vi "MenuActive(Data).vi"(8 "error in (no error)":errorcluster caption="错误输入（无错误）", 10 "菜单引用":refnum<k9>, 11 "PanelDataNode 输入":refnum<class "PanelDataNode.lvclass"> caption="DNL_LabVIEW Object in") -> (0 "error out":errorcluster caption="错误输出", 2 "menu reference out":refnum<k9>, 3 "PanelDataNode 输出":refnum<class "PanelDataNode.lvclass"> caption="DNL_LabVIEW Object out")   [LabVIEW 2013, in "PanelDataNode.lvclass"]
uses:
  PanelDataNode.lvclass
  PanelDataNode.lvclass/PanelDataNode.ctl
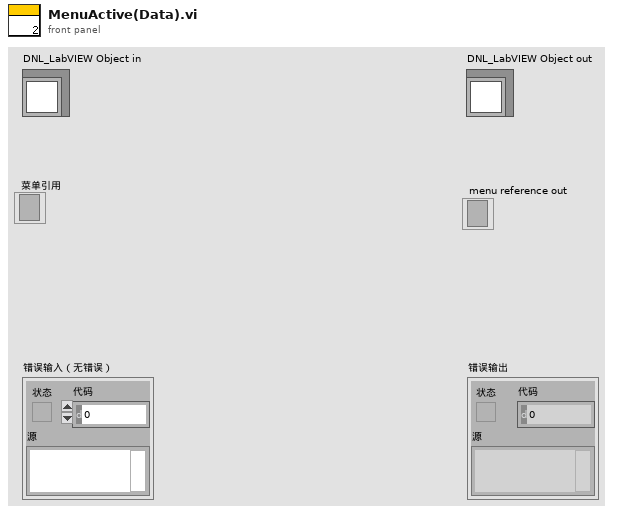
[diagram p1: front panel]
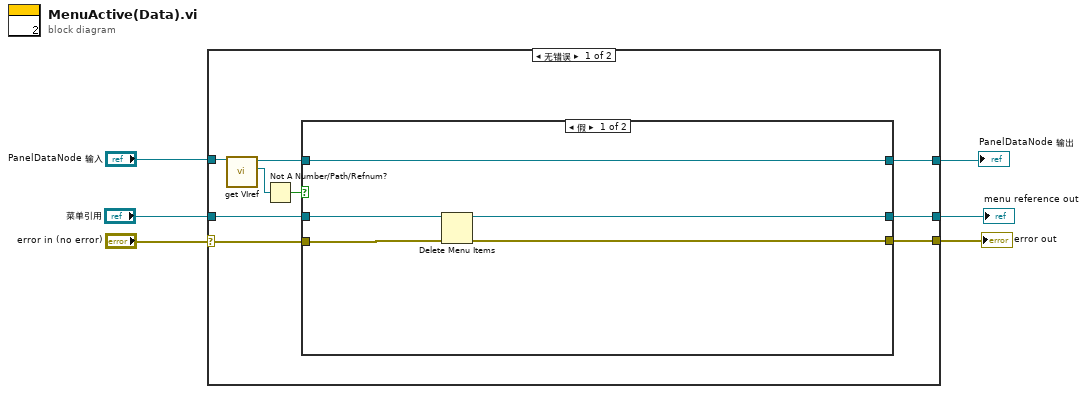
[diagram p0: block diagram]
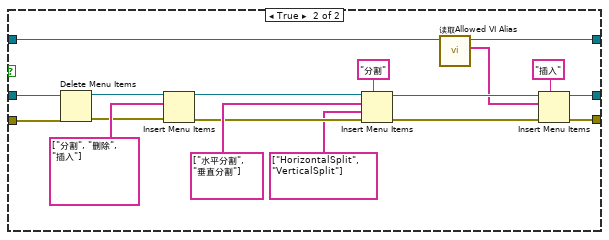
[diagram p2: hidden frame]
diagram:
  n1 = case shown="无错误" "error in (no error)" {
    selector: "error in (no error)" -> [w13 w41]
    tunnel: [w14 w40] -> w5
    tunnel: [w15 w41] -> w4
    tunnel: "PanelDataNode 输入" -> [w10 w40]
    tunnel: "菜单引用" -> [w9 w39]
    tunnel: [w8 w39] -> w1
    frame No Error {
      n2 = call "get VIref.vi"("PanelDataNode输入"=w10) -> ("VI*"=w7:refnum<vi>, "PanelDataNode输出"=w12:refnum<class "PanelDataNode.lvclass">)  [unwired: 8 in, 1 out]
      n3 = Not A Number/Path/Refnum?(number/path/refnum=w7) -> (NaN/Path/Refnum?=w11:bool)
      n4 = case shown="假" w11 {
        tunnel: [w17 w29] -> w15
        tunnel: w12 -> [w20 w27]
        tunnel: [w20 w25] -> w14
        tunnel: w13 -> [w18 w23]
        tunnel: w9 -> [w19 w22]
        tunnel: [w16 w21] -> w8
        frame False {
          n5 = Delete Menu Items(6:w18, 9:w19) -> (0:w17:errorcluster, 3:w16:refnum<k9>)  [unwired: 2 in]
        }
        frame True {
          n6 = Delete Menu Items(6:w23, 9:w22) -> (0:w33:errorcluster, 3:w38:refnum<k9>)  [unwired: 2 in]
          n7 = Insert Menu Items(6:w33, 8:string[] ["分割", "删除", "插入"] ("项名称"), 9:w38) -> (0:w32:errorcluster, 3:w36:refnum<k9>)  [unwired: 3 in, 1 out]
          n8 = Insert Menu Items(5:"分割" ("菜单标识符"), 6:w32, 7:string[] ["HorizontalSplit", "VerticalSplit"] ("项标识符"), 8:string[] ["水平分割", "垂直分割"] ("项名称"), 9:w36) -> (0:w24:errorcluster, 3:w30:refnum<k9>)  [unwired: 1 in, 1 out]
          n9 = call "读取Allowed VI Alias.vi"("PanelDataNode输入"=w27) -> ("Allowed VI Alias"=w26:string[], "PanelDataNode输出"=w25:refnum<class "PanelDataNode.lvclass">)  [unwired: 8 in, 1 out]
          n10 = Insert Menu Items(5:"插入" ("菜单标识符"), 6:w24, 8:w26, 9:w30) -> (0:w29:errorcluster, 3:w21:refnum<k9>)  [unwired: 2 in, 1 out]
        }
      }
    }
    frame Error {
    }
  }
  "error out" <- w4
  "PanelDataNode 输出" <- w5
  "menu reference out" <- w1
